vi "Set Tx Generic Properties.vi"(8 "error in":errorcluster, 10 "session_tx_generic":T1 {"StartMode" items=["FDX_STOP", "FDX_START", "FDX_START_TRG", "FDX_START_TIME"]}, 11 "custom device ref in":T2 format="%.0x") -> (0 "error out":errorcluster, 3 "custom device ref out":T2 format="%.0x")   [LabVIEW 2020, in "AIM ARINC 664 Scripting.lvlib"]
uses:
  AIM ARINC 664 Scripting.lvlib
  <vilib>/NI VeriStand/Custom Device API/Custom Device API.lvlib
  <vilib>/NI VeriStand/Custom Device API/Set Item Property (U32).vi
  Constants.vi
  <vilib>/NI VeriStand/Custom Device API/Custom Device Item Ref.ctl
  Shared/session_tx_generic.ctl
  Import/AIM ARINC 664 Import.lvlib
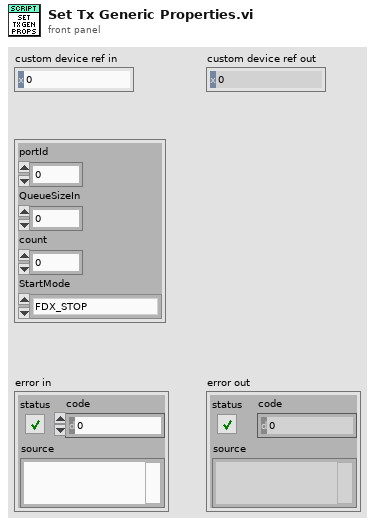
[diagram p1: front panel]
types:
  T1 = typedef "session_tx_generic.ctl" = cluster{"portId":u32, "QueueSizeIn":u32, "count":i32, "StartMode":i32}
  T2 = typedef "Custom Device API.lvlib/Custom Device Item Ref.ctl" = u64
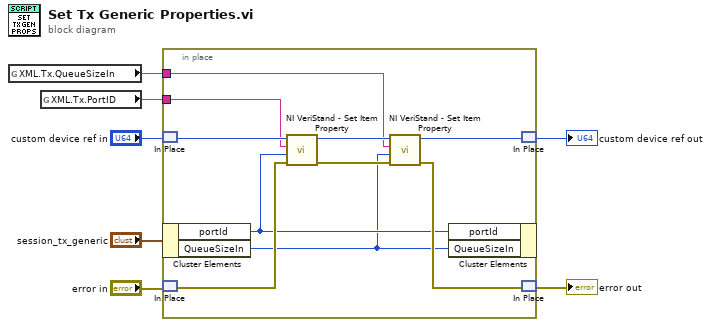
[diagram p0: block diagram]
diagram:
  n1 = global read "Constants.vi" "XML.Tx.QueueSizeIn"() -> (w3:string)
  n2 = global read "Constants.vi" "XML.Tx.PortID"() -> (w2:string)
  n3 = in-place {
    in-place-border: w3 -> [w9]
    in-place-border: w2 -> [w8]
    n4 = in-place-match #1("custom device ref in") -> (w13:T2)
    n5 = in-place-cluster #2("session_tx_generic") -> ("portId"=w15:u32, "QueueSizeIn"=w11:u32)
    n6 = in-place-match #3("error in") -> (w17:errorcluster)
    n7 = call-poly <vilib>:"NI VeriStand - Set Item Property.vi"("error in (no error)"=w17, "Value"=w15, "Property Name"=w8, "Item Ref in"=w13) -> ("error out"=w14:errorcluster, "Item Ref out"=w12:T2)  [unwired: 5 in, 1 out]
    n8 = call-poly <vilib>:"NI VeriStand - Set Item Property.vi"("error in (no error)"=w14, "Value"=w11, "Property Name"=w9, "Item Ref in"=w12) -> ("error out"=w16:errorcluster, "Item Ref out"=w10:T2)  [unwired: 5 in, 1 out]
    n9 = in-place-cluster #2("portId"=w15, "QueueSizeIn"=w11) -> ()  [unwired: 1 out]
    n10 = in-place-match #1(w10) -> (→"custom device ref out":T2)
    n11 = in-place-match #3(w16) -> (→"error out":errorcluster)
  }
